vi "Read GroupChans.vi"(8 "error in (no error)":errorcluster, 11 "ChanGrp in":refnum<class "ChanGrp.lvclass">) -> (0 "error out":errorcluster, 2 "GroupChans":refnum<class "Channel.lvclass">[](array[class]), 3 "ChanGrp out":refnum<class "ChanGrp.lvclass">)   [LabVIEW 2012, in "Configuration Grandmaster.lvlib" / "ChanGrp.lvclass"]
uses:
  ChanGrp.lvclass
  Measurements/Class Channel/Channel.lvclass
  ChanGrp.lvclass/ChanGrp.ctl
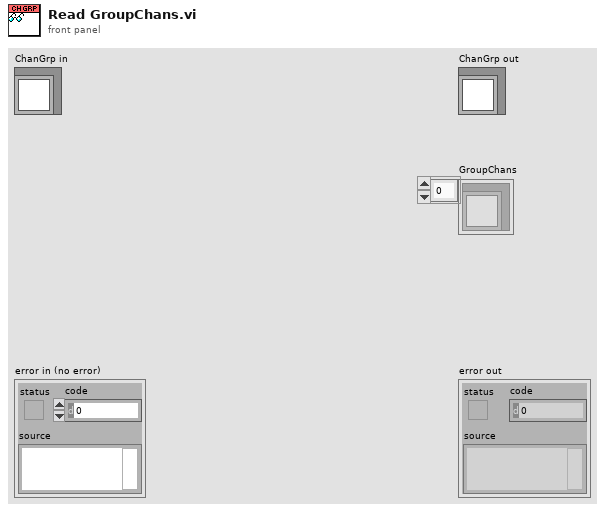
[diagram p1: front panel]
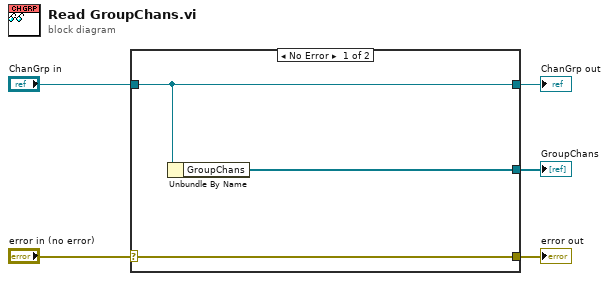
[diagram p0: block diagram]
diagram:
  n1 = case shown="No Error" "error in (no error)" {
    selector: "error in (no error)" -> [w8 w9]
    tunnel: [w8 w9] -> w4
    tunnel: [w7 w10] -> w2
    tunnel: "ChanGrp in" -> [w7 w10]
    tunnel: [w6 _] -> w1
    frame No Error {
      n2 = Unbundle By Name(w7) -> ("GroupChans"=w6:refnum<class "Channel.lvclass">[])
    }
    frame Error {
    }
  }
  "error out" <- w4
  "ChanGrp out" <- w2
  "GroupChans" <- w1
